vi "Seek Locate Destory.vi"(8 "String to Delete":string, 10 "Input String Array":string[](array[string])) -> (1 "Output Array":string[](array[string]))   [LabVIEW 2014]
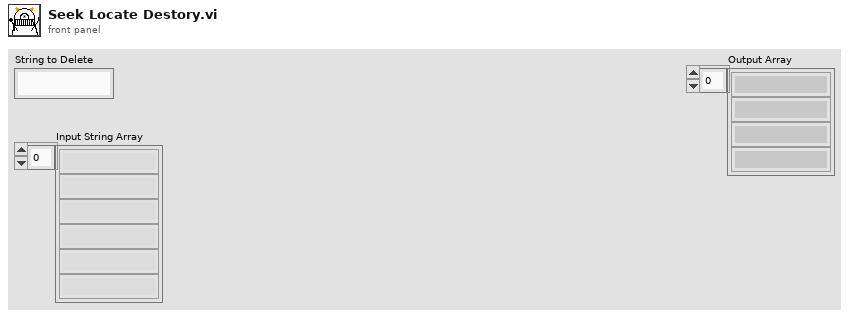
[diagram p1: front panel]
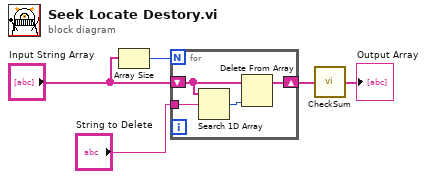
[diagram p0: block diagram]
diagram:
  n1 = Array Size(array="Input String Array") -> (size(s)=w4:i32)
  n2 = for {
    N: w4 -> [_]
    tunnel: "String to Delete" -> [w8]
    shift-right: [w9] -> w2
    shift-left: "Input String Array" -> [w7]
    n3 = Search 1D Array(1D array=w7, element=w8) -> (index of element=w6:i32)  [unwired: 1 in]
    n4 = Delete From Array(array=w7, index=w6) -> (array with subset deleted=w9:string[])  [unwired: 1 in, 1 out]
  }
  n5 = call "CheckSum.vi"("Input String Array"=w2) -> ("Output String Array"=→"Output Array":string[])
